vi "Write Record Data.vi"(8 "Error In (no error)":errorcluster, 10 "Record":variant, 11 "Expenses Tracker Subcategory In":refnum<class "Expenses Tracker Subcategory.lvclass">) -> (0 "Error Out":errorcluster, 3 "Expenses Tracker Subcategory Out":refnum<class "Expenses Tracker Subcategory.lvclass">)   [LabVIEW 2023, in "Expenses Tracker Subcategory.lvclass"]
uses:
  Expenses Tracker Subcategory.lvclass
  Ctrls/Subcategory.ctl
  Expenses Tracker Subcategory.lvclass/Expenses Tracker Subcategory.ctl
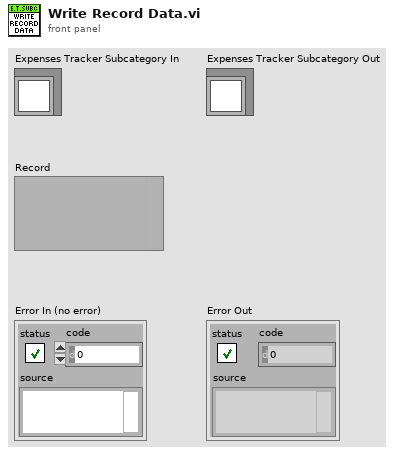
[diagram p1: front panel]
types:
  T1 = typedef "Expenses Tracker Subcategory.lvclass/Subcategory.ctl" = cluster{"ID":u32, "Name":string, "Category":u32}
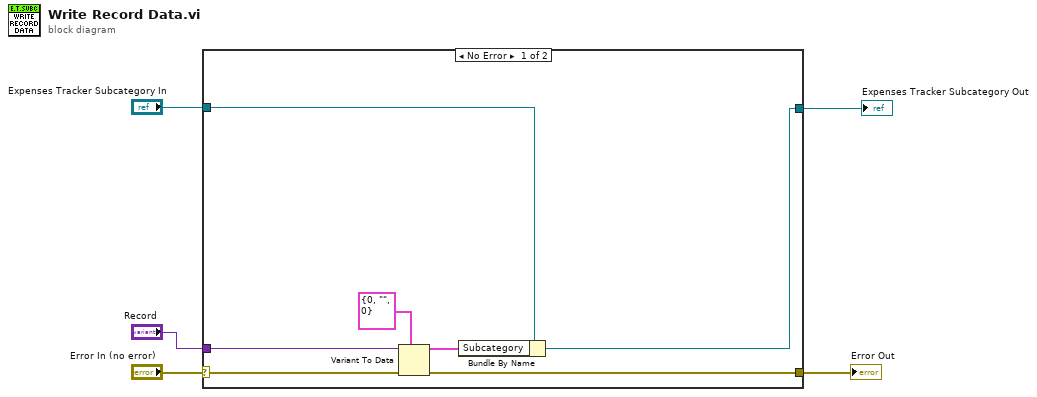
[diagram p0: block diagram]
diagram:
  n1 = case shown="No Error" "Error In (no error)" {
    selector: "Error In (no error)" -> [w10 w14]
    tunnel: [w8 w14] -> w4
    tunnel: [w7 w13] -> w3
    tunnel: "Expenses Tracker Subcategory In" -> [w6 w13]
    tunnel: "Record" -> [w12 _]
    frame No Error {
      n2 = Variant To Data(error in=w10, type=T1 {"ID"=0, "Name"="", "Category"=0} ("Subcategory"), Variant=w12) -> (data=w11:T1, error out=w8:errorcluster)
      n3 = Bundle By Name(cluster=w6, "Subcategory"=w11) -> (w7:refnum<class "Expenses Tracker Subcategory.lvclass">)
    }
    frame Error {
    }
  }
  "Error Out" <- w4
  "Expenses Tracker Subcategory Out" <- w3
